vi "Break Blob Lease.vi"(6 "Break period in seconds (-1: none)":i32=-1, 8 "error in (no error)":errorcluster, 9 "Blob":string, 10 "Container":string, 11 "Azure Session in":refnum<class "Session.lvclass">) -> (0 "error out":errorcluster, 3 "Azure Session out":refnum<class "Session.lvclass">)   [LabVIEW 2015, in "NI_Azure_Blob.lvlib"]
doc: "End the blob lease but ensure that another client cannot acquire a new lease until the current lease period has expired."
uses:
  NI_Azure_Blob.lvlib
  Core/Session/Session.lvclass
  Core/Name Value Pair.ctl
  Lease Action.ctl
  Core/Session/Session.lvclass/Session.ctl
  Core/Session/Write Request Headers.vi
  Core/Session/Write Request Parameters.vi
  Core/Session/Write HTTP Verb.vi
  Core/Session/Write URL Suffix.vi
  Strings Global.vi
  Core/NI_Azure_Core.lvlib
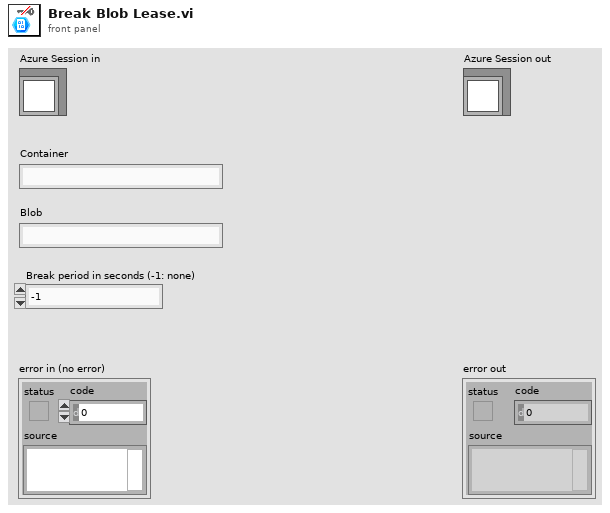
[diagram p1: front panel]
types:
  T1 = typedef "NI_Azure_Blob.lvlib/Lease Action.ctl" = enum16{"acquire", "renew", "change", "release", "break"}
  T2 = typedef "NI_Azure_Core.lvlib/Name Value Pair.ctl" = cluster{"name":string, "value":string}
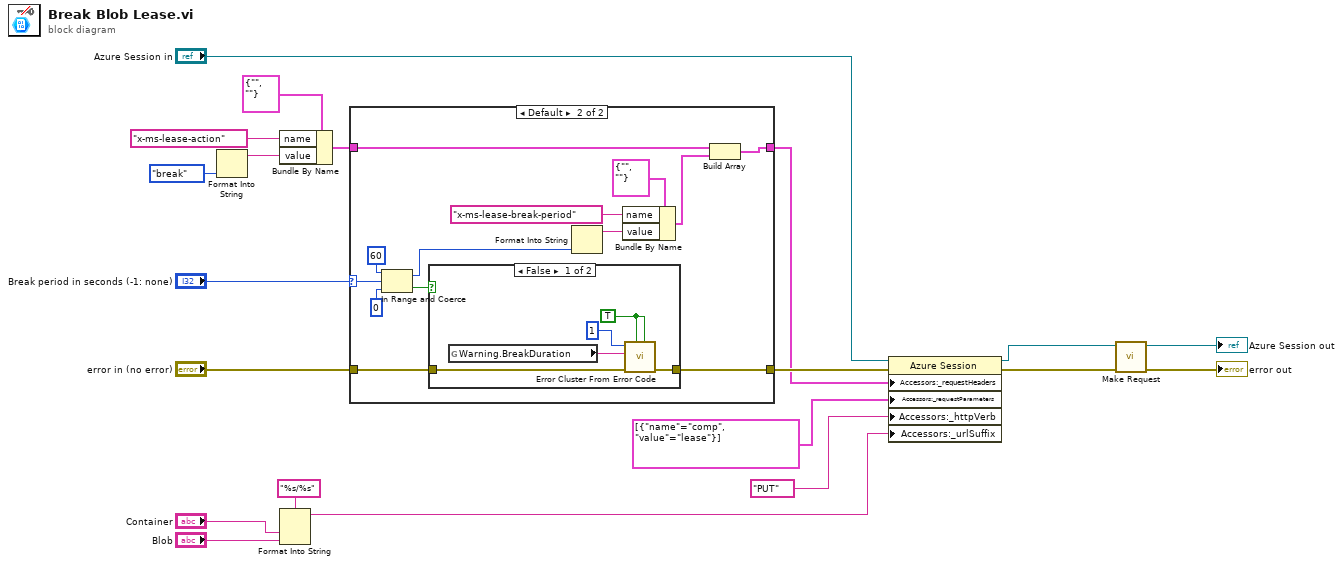
[diagram p0: block diagram]
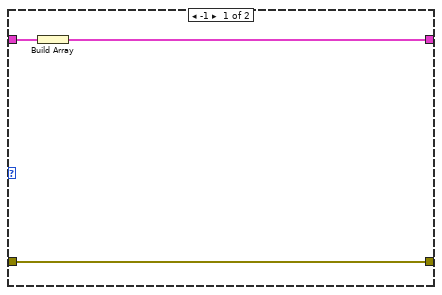
[diagram p2: hidden frame]
diagram:
  n1 = Format Into String(Lease_Action."break" ("Lease action")) -> (resulting string=w14:string)  [unwired: 3 in, 1 out]
  n2 = Bundle By Name(cluster=T2 {"name"="", "value"=""} ("Cluster"), "name"="x-ms-lease-action" ("header"), "value"=w14) -> (w8:T2)
  n3 = Format Into String(format string="%s/%s", "Container", "Blob") -> (resulting string=w1:string)  [unwired: 2 in, 1 out]
  n4 = case shown="Default" "Break period in seconds (-1: none)" {
    selector: "Break period in seconds (-1: none)" -> [_ w31]
    tunnel: [w21 w24] -> w4
    tunnel: "error in (no error)" -> [w23 w33]
    tunnel: [w23 w32] -> w10
    tunnel: w8 -> [w22 w26]
    frame -1 {
      n5 = Build Array(w22) -> (w21:T2[])
    }
    frame Default {
      n6 = In Range and Coerce(upper limit=60, x=w31, lower limit=0) -> (coerced(x)=w30:i32, In Range?=w27:bool)
      n7 = case shown="False" w27 {
        tunnel: w33 -> [w40 w42]
        tunnel: [w39 w42] -> w32
        frame False {
          w41 = TRUE ("show call chain? (False)")
          n8 = global read "Strings Global.vi" "Warning.BreakDuration"() -> (w37:string)
          n9 = call <vilib>:"Error Cluster From Error Code.vi"("is warning? (False)"=w41, "show call chain? (False)"=w41, "error in (no error)"=w40, "error message (\"\")"=w37, "error code (0)"=1) -> ("error out"=w39:errorcluster)  [unwired: 4 in]
        }
        frame True {
        }
      }
      n10 = Format Into String(w30) -> (resulting string=w35:string)  [unwired: 3 in, 1 out]
      n11 = Bundle By Name(cluster=T2 {"name"="", "value"=""} ("Cluster"), "name"="x-ms-lease-break-period" ("header"), "value"=w35) -> (w25:T2)
      n12 = Build Array(w26, w25) -> (w24:T2[])
    }
  }
  n13 = property class="Azure Session"(reference="Azure Session in", error in=w10, "Accessors:_requestHeaders"=w4, "Accessors:_requestParameters"=T2[] [{"name"="comp", "value"="lease"}] ("request parameters"), "Accessors:_httpVerb"="PUT" ("HTTP-Verb"), "Accessors:_urlSuffix"=w1) -> (reference out=w5:refnum<class "Session.lvclass">, error out=w7:errorcluster)
  n14 = call "Make Request.vi"("error in (no error)"=w7, "Session in"=w5) -> ("error out"=→"error out":errorcluster, "Session out"=→"Azure Session out":refnum<class "Session.lvclass">)  [unwired: 7 in, 1 out]
